vi "ExpVar UpdLoop_ExpCondition.vi"(8 "error in (no error)":errorcluster, 11 "NewExpVar in":refnum<class "ExpVar.lvclass">) -> (0 "error out":errorcluster, 3 "NewExpVar out":refnum<class "ExpVar.lvclass">)   [LabVIEW 2018, in "ExpVar.lvclass"]
uses:
  ExpVar.lvclass
  ExpVar.lvclass/ExpVar.ctl
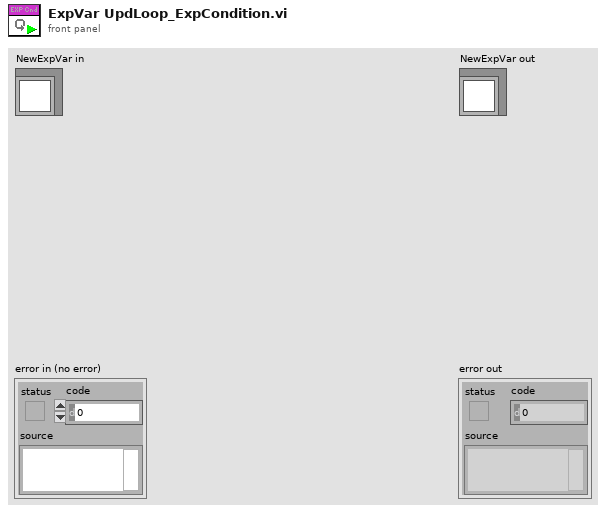
[diagram p1: front panel]
types:
  T1 = cluster{cluster{"Label":string, "Value":variant}[]}[]
  T2 = cluster{cluster{"Label":string, "Value":variant}[]}
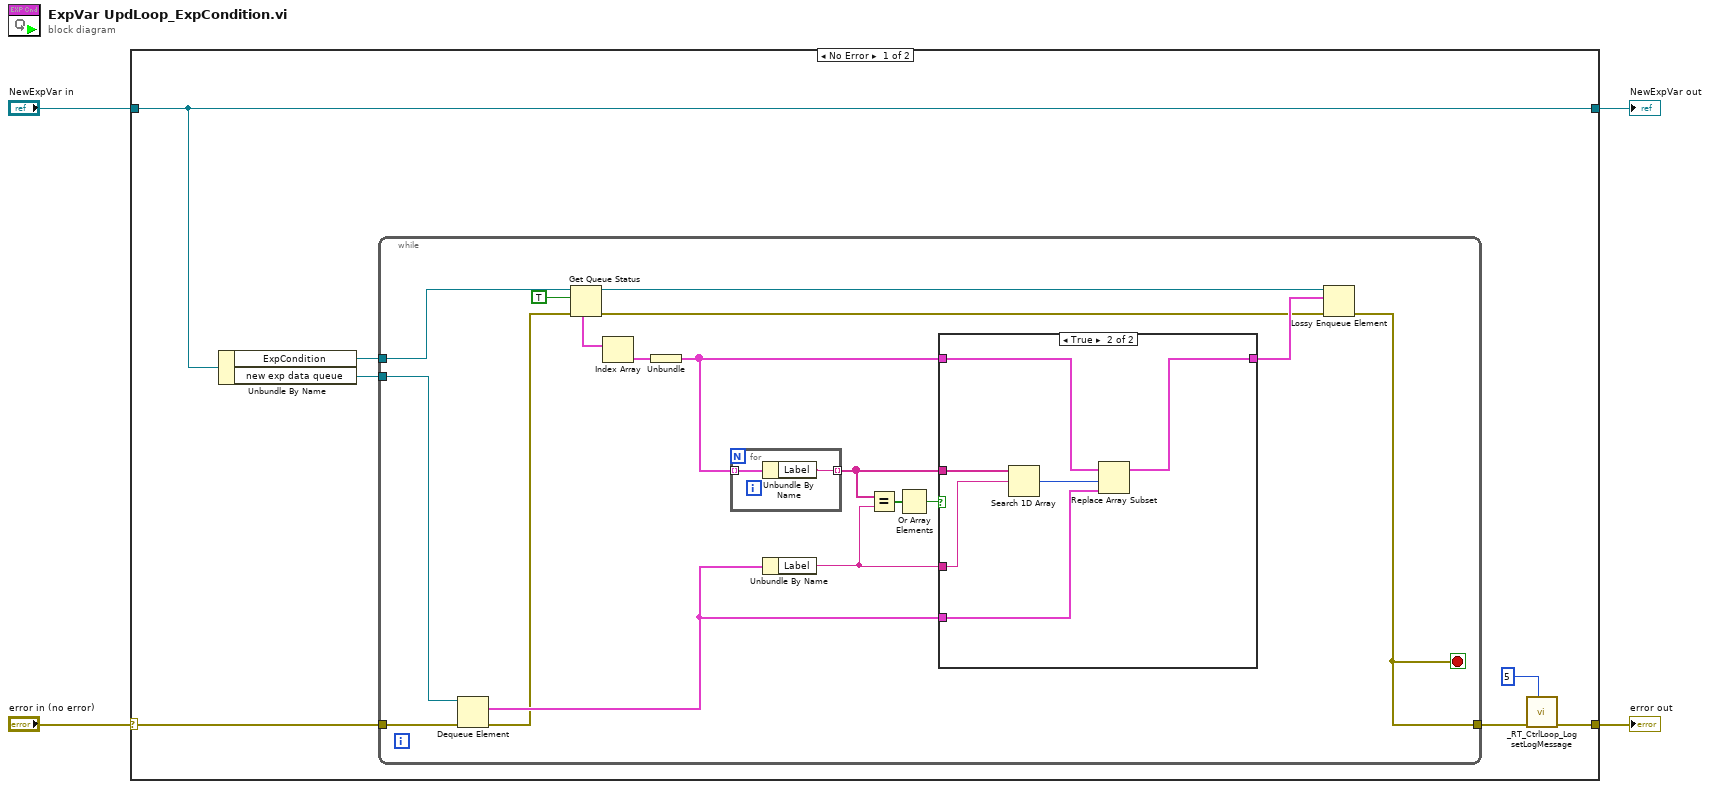
[diagram p0: block diagram]
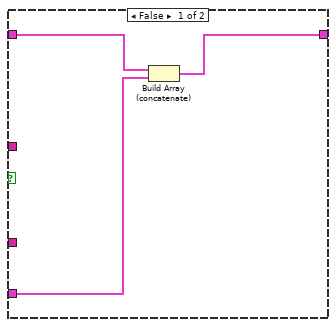
[diagram p2: hidden frame]
diagram:
  n1 = case shown="No Error" "error in (no error)" {
    selector: "error in (no error)" -> [w8 w41]
    tunnel: [w5 w41] -> w3
    tunnel: [w11 w40] -> w1
    tunnel: "NewExpVar in" -> [w11 w40]
    frame No Error {
      n2 = Unbundle By Name(w11) -> ("ExpCondition"=w9:refnum<queue>, "new exp data queue"=w10:refnum<queue>)
      n3 = while {
        tunnel: w10 -> [w28]
        tunnel: w9 -> [w22]
        tunnel: w8 -> [w13]
        tunnel: [w12] -> w6
        stop <- w12 stop-if-true
        n4 = Dequeue Element(queue=w28, error in (no error)=w13) -> (element=w26:cluster{"Label":string, "Value":variant}, error out=w14:errorcluster)  [unwired: 1 in, 2 out]
        n5 = Get Queue Status(queue=w22, return elements? (F)=TRUE, error in (no error)=w14) -> (queue out=w17:refnum<queue>, error out=w15:errorcluster, elements=w19:T1)  [unwired: 5 out]
        n6 = Index Array(array=w19) -> (element=w20:T2)  [unwired: 1 in]
        n7 = Unbundle(w20) -> (w18:cluster{"Label":string, "Value":variant}[])
        n8 = for {
          tunnel: w18 -> [w39] mode=indexing
          tunnel: [w38] -> w23 mode=indexing
          n9 = Unbundle By Name(w39) -> ("Label"=w38:string)
        }
        n10 = Unbundle By Name(w26) -> ("Label"=w27:string)
        n11 = Equal?(x=w23, y=w27) -> (x = y?=w25:bool[])
        n12 = Or Array Elements(Boolean array=w25) -> (logical OR=w24:bool)
        n13 = case shown="True" w24 {
          tunnel: w23 -> [_ w37]
          tunnel: w27 -> [_ w36]
          tunnel: w18 -> [w31 w35]
          tunnel: w26 -> [w29 w34]
          tunnel: [w30 w32] -> w16
          frame False {
            n14 = Build Array (concatenate)(w31, w29) -> (w30:cluster{"Label":string, "Value":variant}[])
          }
          frame True {
            n15 = Search 1D Array(1D array=w37, element=w36) -> (index of element=w33:i32)  [unwired: 1 in]
            n16 = Replace Array Subset(array=w35, new element=w34, index=w33) -> (w32:cluster{"Label":string, "Value":variant}[])
          }
        }
        n17 = Lossy Enqueue Element(queue=w17, element=w16, error in (no error)=w15) -> (error out=w12:errorcluster)  [unwired: 3 out]
      }
      n18 = call "_RT_CtrlLoop_Log setLogMessage.vi"("system type"=u16 5 ("N1"), "error in"=w6) -> ("error out"=w5:errorcluster)  [unwired: 8 in, 1 out]
    }
    frame Error {
    }
  }
  "error out" <- w3
  "NewExpVar out" <- w1
